vi "Read RandomValue.vi"(8 "error in (no error)":errorcluster, 11 "Data in":refnum<class "Data.lvclass">) -> (0 "error out":errorcluster, 2 "RandomValue":dbl, 3 "Data out":refnum<class "Data.lvclass">)   [LabVIEW 2014, in "Data.lvclass"]
uses:
  Data.lvclass
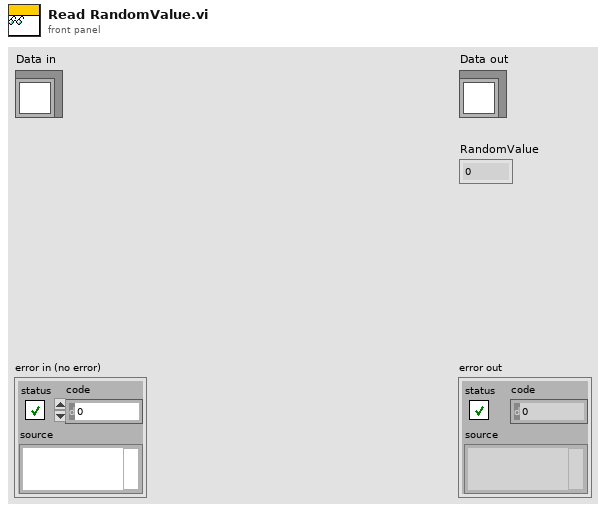
[diagram p1: front panel]
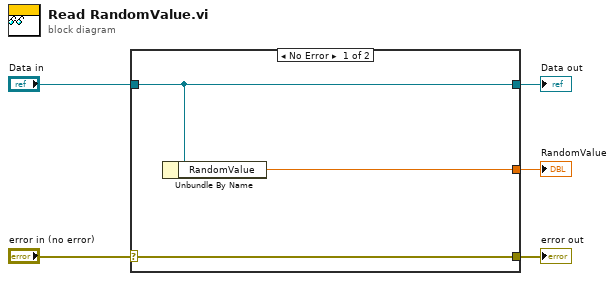
[diagram p0: block diagram]
diagram:
  n1 = case shown="No Error" "error in (no error)" {
    selector: "error in (no error)" -> [w8 w9]
    tunnel: [w8 w9] -> w4
    tunnel: [w7 w10] -> w2
    tunnel: "Data in" -> [w7 w10]
    tunnel: [w6 _] -> w1
    frame No Error {
      n2 = Unbundle By Name(w7) -> ("RandomValue"=w6:dbl)
    }
    frame Error {
    }
  }
  "error out" <- w4
  "Data out" <- w2
  "RandomValue" <- w1
